vi "Flush.vi"(0 "object in":refnum<class "Application.lvclass">=refnum, 2 "Wait (s)":dbl=2.0, 5 "error in (no error)":errorcluster) -> (14 "object out":refnum<class "Application.lvclass">, 19 "error out":errorcluster)   [LabVIEW 2023, in "Application.lvclass"]
uses:
  Application.lvclass
  Valve_class/Valve.lvclass
  CetoniPump_class/CetoniPump.lvclass
  Hamamatsu_simulated_class/Hamamatsu_simulated.lvclass
  AD2_SDK_class/AD2_SDK.lvclass
  AD2_MSO_SDK_class/AD2_MSO_SDK.lvclass
  AD2_WFG_SDK_class/AD2_WFG_SDK.lvclass
  AD2_DO_SDK_class/AD2_DO_SDK.lvclass
  Valve_Sim_class/Valve_Sim.lvclass
  Cetoni_Simulated_class/Cetoni_Simulated.lvclass
  Prior_Zmotor_class/Prior_Zmotor.lvclass
  Experiment2_class/Experiment2.lvclass
  ExperimentSeries2_class/ExperimentSeries2.lvclass
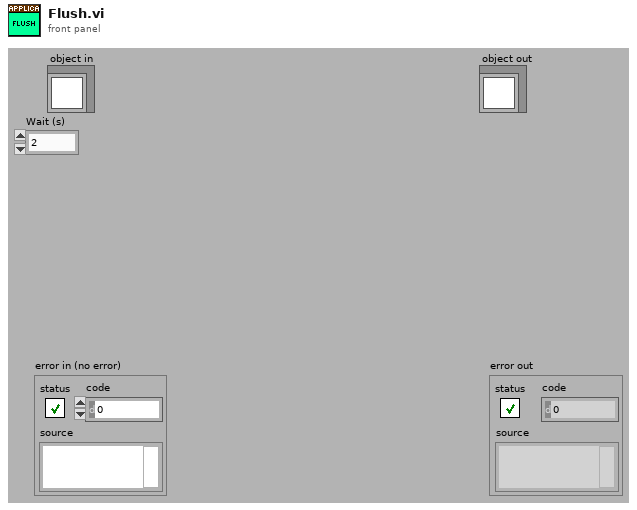
[diagram p1: front panel]
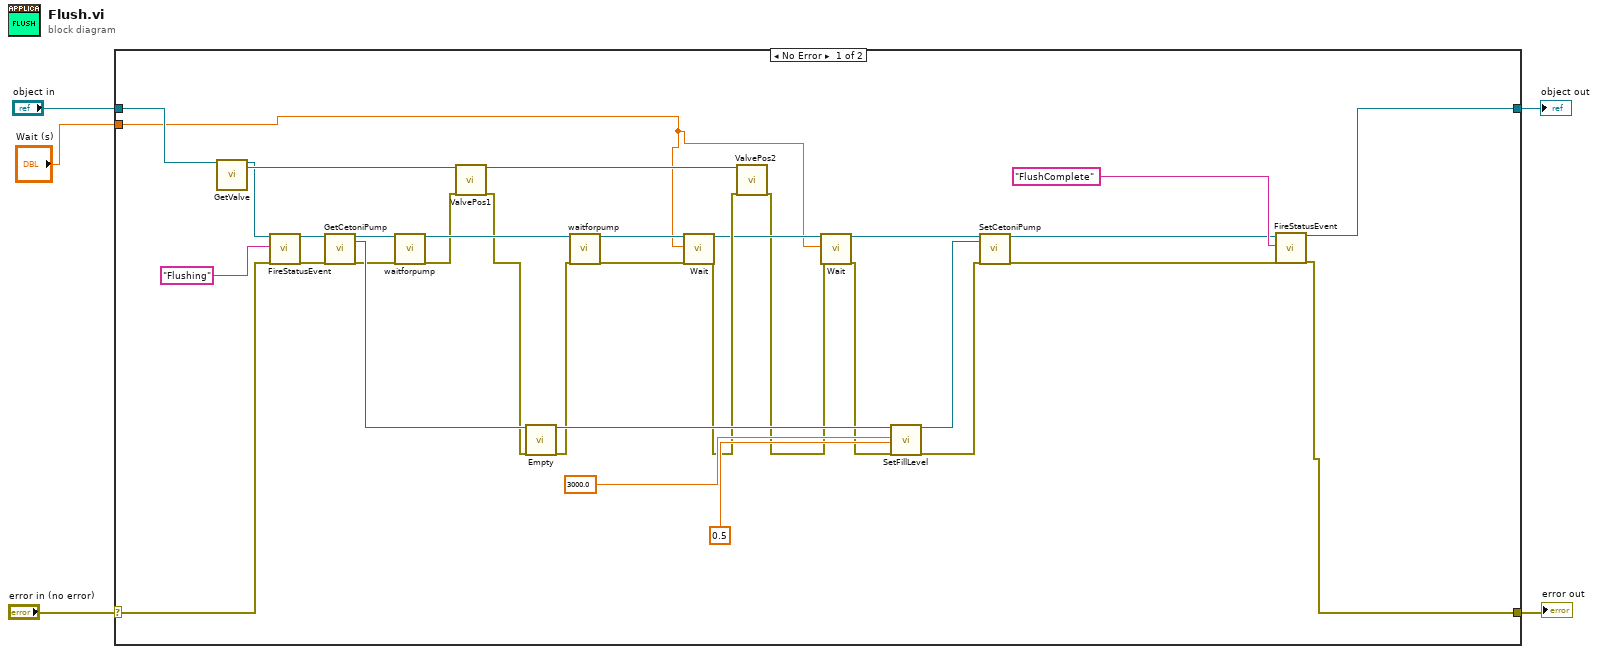
[diagram p0: block diagram]
diagram:
  n1 = case shown="No Error" "error in (no error)" {
    selector: "error in (no error)" -> [w30 w40]
    tunnel: [w29 w40] -> w4
    tunnel: [w9 w39] -> w2
    tunnel: "object in" -> [w7 w39]
    tunnel: "Wait (s)" -> [w6 _]
    frame No Error {
      n2 = call-dynamic "GetValve.vi"("object in"=w7) -> ("object out"=w8:refnum<class "Application.lvclass">, "Valve"=w28:refnum<class "Valve.lvclass">)  [unwired: 16 in, 1 out]
      n3 = call-dynamic "FireStatusEvent.vi"("object in"=w8, "Status"="Flushing", "error in (no error)"=w30) -> ("object out"=w37:refnum<class "Application.lvclass">, "error out"=w27:errorcluster)  [unwired: 15 in]
      n4 = call-dynamic "GetCetoniPump.vi"("object in"=w37, "error in (no error)"=w27) -> ("object out"=w34:refnum<class "Application.lvclass">, "CetoniPump"=w35:refnum<class "CetoniPump.lvclass">, "error out"=w26:errorcluster)  [unwired: 15 in]
      n5 = call-dynamic "waitforpump.vi"("object in"=w34, "error in (no error)"=w26) -> ("object out"=w24:refnum<class "Application.lvclass">, "error out"=w12:errorcluster)  [unwired: 15 in, 1 out]
      n6 = call-dynamic "ValvePos1.vi"("object in"=w28, "error in (no error)"=w12) -> ("object out"=w22:refnum<class "Valve.lvclass">, "error out"=w11:errorcluster)  [unwired: 16 in]
      n7 = call-dynamic "Empty.vi"("object in"=w35, "error in (no error)"=w11) -> ("object out"=w36:refnum<class "CetoniPump.lvclass">, "error out"=w25:errorcluster)  [unwired: 16 in]
      n8 = call-dynamic "waitforpump.vi"("object in"=w24, "error in (no error)"=w25) -> ("object out"=w23:refnum<class "Application.lvclass">, "error out"=w17:errorcluster)  [unwired: 15 in, 1 out]
      n9 = call-dynamic "Wait.vi"("object in"=w23, "Wait (s)"=w6, "error in (no error)"=w17) -> ("object out"=w16:refnum<class "Application.lvclass">, "error out"=w21:errorcluster)  [unwired: 15 in]
      n10 = call-dynamic "ValvePos2.vi"("object in"=w22, "error in (no error)"=w21) -> ("error out"=w14:errorcluster)  [unwired: 16 in, 1 out]
      n11 = call-dynamic "Wait.vi"("object in"=w16, "Wait (s)"=w6, "error in (no error)"=w14) -> ("object out"=w15:refnum<class "Application.lvclass">, "error out"=w13:errorcluster)  [unwired: 15 in]
      n12 = call-dynamic "SetFillLevel.vi"("object in"=w36, "Flow"=3000.0 ("Level(ml)"), "Level(ml)"=0.5 ("Flow"), "error in (no error)"=w13) -> ("object out"=w19:refnum<class "CetoniPump.lvclass">, "error out"=w18:errorcluster)  [unwired: 14 in]
      n13 = call-dynamic "SetCetoniPump.vi"("object in"=w15, "CetoniPump"=w19, "error in (no error)"=w18) -> ("object out"=w20:refnum<class "Application.lvclass">, "error out"=w10:errorcluster)  [unwired: 15 in]
      n14 = call-dynamic "FireStatusEvent.vi"("object in"=w20, "Status"="FlushComplete", "error in (no error)"=w10) -> ("object out"=w9:refnum<class "Application.lvclass">, "error out"=w29:errorcluster)  [unwired: 15 in]
    }
    frame Error {
    }
  }
  "error out" <- w4
  "object out" <- w2
